vi "Get Bias Voltage.vi"(8 "error in (no error)":errorcluster, 9 "Channel":i32, 11 "VoltageUpdate in":refnum<class "VoltageUpdate.lvclass">) -> (0 "error out":errorcluster, 2 "Bias Voltage (V)":dbl, 3 "VoltageUpdate out":refnum<class "VoltageUpdate.lvclass">)   [LabVIEW 2016, in "VoltageUpdate.lvclass"]
uses:
  VoltageUpdate.lvclass
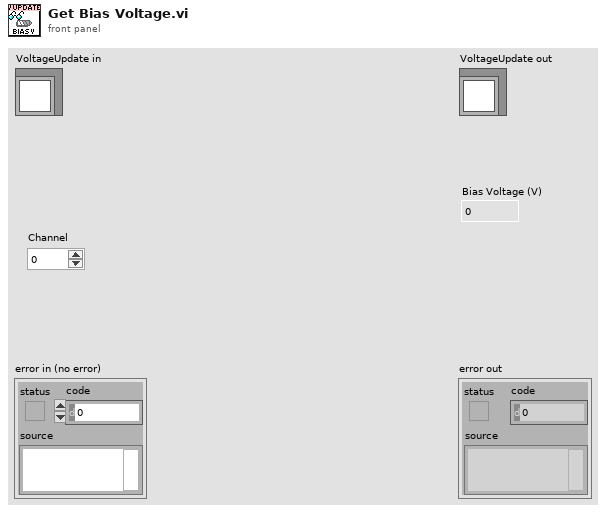
[diagram p1: front panel]
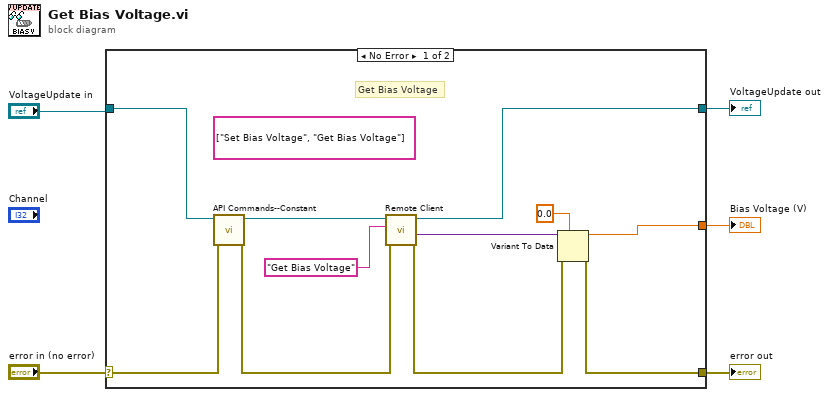
[diagram p0: block diagram]
diagram:
  n1 = case shown="No Error" "error in (no error)" {
    selector: "error in (no error)" -> [w16 w18]
    tunnel: [w8 w18] -> w3
    tunnel: [w12 w17] -> w2
    tunnel: "VoltageUpdate in" -> [w13 w17]
    tunnel: [w7 _] -> w1
    frame No Error {
      (unwired) string[] ["Set Bias Voltage", "Get Bias Voltage"] ("Array")
      # "Get Bias Voltage"
      n2 = call "API Commands--Constant.vi"("error in (no error)"=w16, "VoltageUpdate in"=w13) -> ("error out"=w15:errorcluster, "VoltageUpdate out"=w14:refnum<class "VoltageUpdate.lvclass">)  [unwired: 7 in, 1 out]
      n3 = call-dynamic "Remote Client.vi"("error in (no error)"=w15, "Command"="Get Bias Voltage", "Instrument in"=w14) -> ("error out"=w9:errorcluster, "Data out"=w10:variant, "Instrument out"=w12:refnum<class "VoltageUpdate.lvclass">)  [unwired: 5 in, 1 out]
      n4 = Variant To Data(error in=w9, type=0.0 ("Bias Voltage (V)"), Variant=w10) -> (data=w7:dbl, error out=w8:errorcluster)
    }
    frame Error {
    }
  }
  "error out" <- w3
  "VoltageUpdate out" <- w2
  "Bias Voltage (V)" <- w1
